vi "E364X Configure Output.vi"(8 "Error In":errorcluster, 9 "Current Limit (0.0 Amps)":dbl format="%.2p", 10 "Level (0.0 Volts)":dbl, 11 "VISA resource In":refnum<visa-resource-name>) -> (0 "Error Out":errorcluster, 3 "VISA resource Out":refnum<visa-resource-name>)   [LabVIEW 2017]
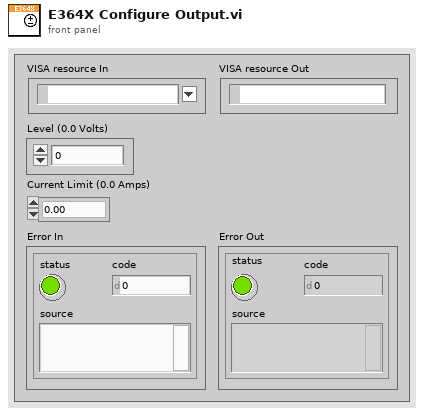
[diagram p1: front panel]
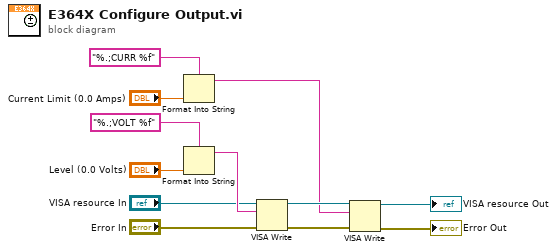
[diagram p0: block diagram]
diagram:
  n1 = Format Into String(format string="%.;CURR %f", "Current Limit (0.0 Amps)") -> (resulting string=w1:string)  [unwired: 2 in, 1 out]
  n2 = Format Into String(format string="%.;VOLT %f", "Level (0.0 Volts)") -> (resulting string=w10:string)  [unwired: 2 in, 1 out]
  n3 = VISA Write(VISA resource name="VISA resource In", write buffer=w10, error in (no error)="Error In") -> (VISA resource name out=w7:refnum<visa-resource-name>, error out=w6:errorcluster)  [unwired: 1 out]
  n4 = VISA Write(VISA resource name=w7, write buffer=w1, error in (no error)=w6) -> (VISA resource name out=→"VISA resource Out":refnum<visa-resource-name>, error out=→"Error Out":errorcluster)  [unwired: 1 out]
